vi "controlRealtimeInputStepsPerPulse.vi"(7 "Set":bool, 8 "error in":errorcluster, 9 "Steps in":i32, 10 "axis in":u8, 11 "connection ID":refnum<k5>) -> (0 "error out":errorcluster, 1 "Steps out":i32, 2 "axis out":u8, 3 "connection ID":refnum<k5>)   [LabVIEW 2016]
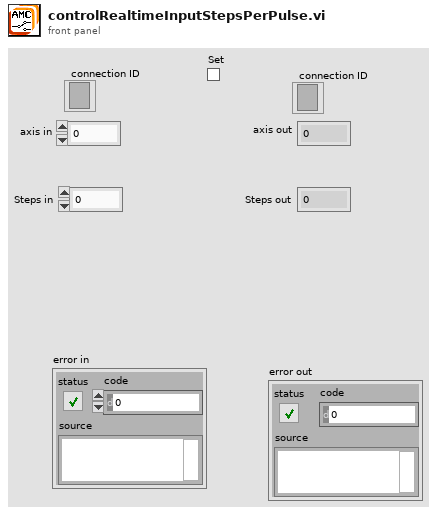
[diagram p1: front panel]
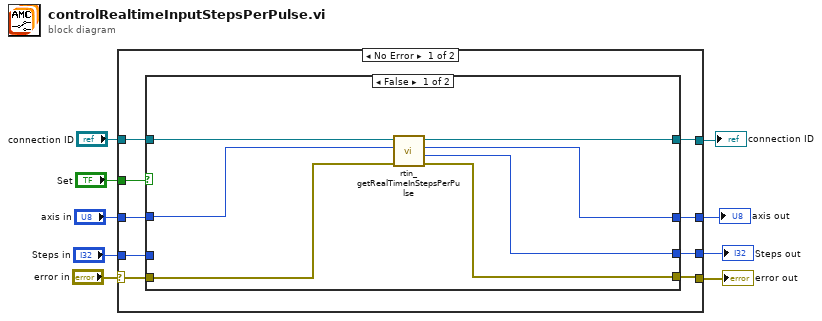
[diagram p0: block diagram]
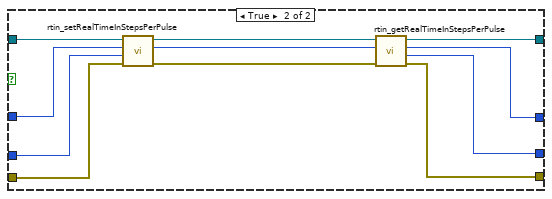
[diagram p2: hidden frame]
diagram:
  n1 = case shown="No Error" "error in" {
    selector: "error in" -> [w10 w39]
    tunnel: "axis in" -> [w16 w38]
    tunnel: [w11 w39] -> w8
    tunnel: [w13 w38] -> w7
    tunnel: "Set" -> [w17 _]
    tunnel: [w14 w37] -> w5
    tunnel: "connection ID" -> [w18 w37]
    tunnel: "Steps in" -> [w15 w40]
    tunnel: [w12 w40] -> w2
    frame No Error {
      n2 = case shown="False" w17 {
        tunnel: [w24 w30] -> w14
        tunnel: w18 -> [w25 w36]
        tunnel: w16 -> [w23 w34]
        tunnel: [w22 w27] -> w13
        tunnel: [w20 w31] -> w11
        tunnel: [w21 w26] -> w12
        tunnel: w15 -> [_ w33]
        tunnel: w10 -> [w19 w35]
        frame False {
          n3 = call "rtin_getRealTimeInStepsPerPulse.vi"("error in"=w19, "axis"=w23, "connection ID"=w25) -> ("error out"=w20:errorcluster, "steps"=w21:i32, "axis_out"=w22:i32, "connection ID"=w24:refnum<k5>)  [unwired: 5 in]
        }
        frame True {
          n4 = call "rtin_setRealTimeInStepsPerPulse.vi"("error in"=w35, "steps"=w33, "axis"=w34, "connection ID"=w36) -> ("error out"=w32:errorcluster, "axis_out"=w28:i32, "connection ID"=w29:refnum<k5>)  [unwired: 5 in]
          n5 = call "rtin_getRealTimeInStepsPerPulse.vi"("error in"=w32, "axis"=w28, "connection ID"=w29) -> ("error out"=w31:errorcluster, "steps"=w26:i32, "axis_out"=w27:i32, "connection ID"=w30:refnum<k5>)  [unwired: 5 in]
        }
      }
    }
    frame Error {
    }
  }
  "error out" <- w8
  "axis out" <- w7
  "connection ID" <- w5
  "Steps out" <- w2
